vi "tkrsa6100 Quote Stripper.vi"(11 "Input String":string) -> (3 "Output String":string)   [LabVIEW 2020, in "Library Instrument & Equipement.lvlib" / "Library Spectrum Analyser.lvlib"]
uses:
  Library Spectrum Analyser.lvlib
panel:
  # "Quote Stripper"
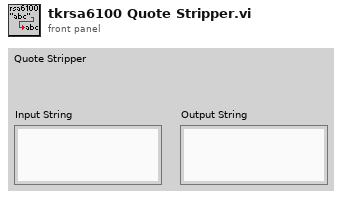
[diagram p1: front panel]
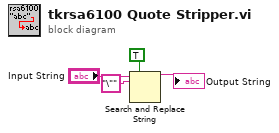
[diagram p0: block diagram]
diagram:
  n1 = Search and Replace String(replace all?=TRUE ("replace all? (F)"), input string="Input String", search string="\"") -> (result string=→"Output String":string)  [unwired: 1 in, 7 out]
